vi "QueryFirst.vi"(6 "commandTimeout in":i32=-1, 7 "CommandType":i32(ring)=-1 items=["Text"=1, "StoredProcedure"=4, "TableDirect"=512], 8 "error in (no error)":errorcluster, 9 "DynamicParameters in":refnum<class "DynamicParameters.lvclass">, 10 "sql":string, 11 "SqlMapper in":refnum<class "DapperMapper.lvclass">) -> (0 "error out":errorcluster, 2 "Value":variant, 3 "SqlMapper out":refnum<class "DapperMapper.lvclass">)   [LabVIEW 2020, in "ORM_Dapper.lvlib" / "DapperMapper.lvclass"]
uses:
  DapperMapper.lvclass
  C:/Program Files/National Instruments/LabVIEW 2020/vi.lib/Viviota/shared/ORM.lvlibp/ORM/SqlMapper/SqlMapper.lvclass
  <vilib>/Viviota/shared/ORM.lvlibp/ORM/DynamicParameters/DynamicParameters.lvclass
  DapperParameters/DapperParameters.lvclass
  DapperRow/DapperRow.lvclass
  DapperParameters/DapperParameters.lvclass/DapperParameters.ctl
  C:/Viviota/Projects/R&D/LabVIEW_ORM/source/src/libraries/dapper/Dapper.dll
  libraries/dapper/Dapper.dll
  <vilib>/Viviota/shared/ORM.lvlibp/ORM/SqlMapper/Read DbConnection.vi
  <vilib>/Viviota/shared/ORM.lvlibp/ORM/DbConnection/Read connection.vi
  <vilib>/Viviota/shared/ORM.lvlibp/ORM/DbConnection/Read transaction.vi
  <vilib>/Viviota/shared/ORM.lvlibp/ORM/DbConnection/DbConnection.lvclass
  System.Data
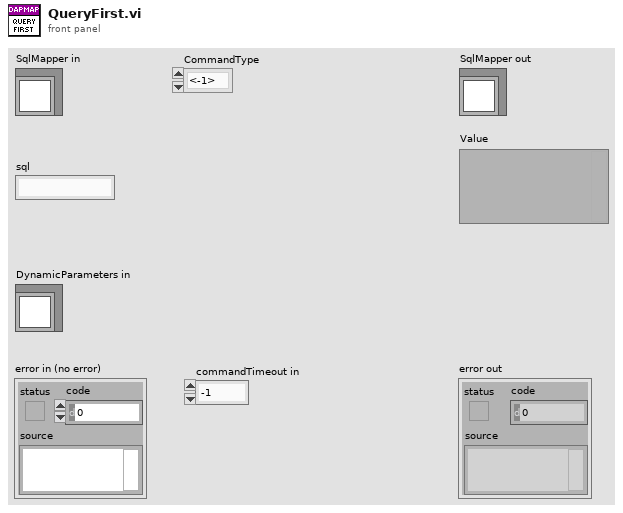
[diagram p1: front panel]
types:
  T1 = typedef "ORM_Dapper.lvlib/dapper_dynamicparameters_ref.ctl" = refnum<k24>
  T2 = typedef "ORM_Dapper.lvlib/dapper_sqlmapper_ref.ctl" = refnum<k24>
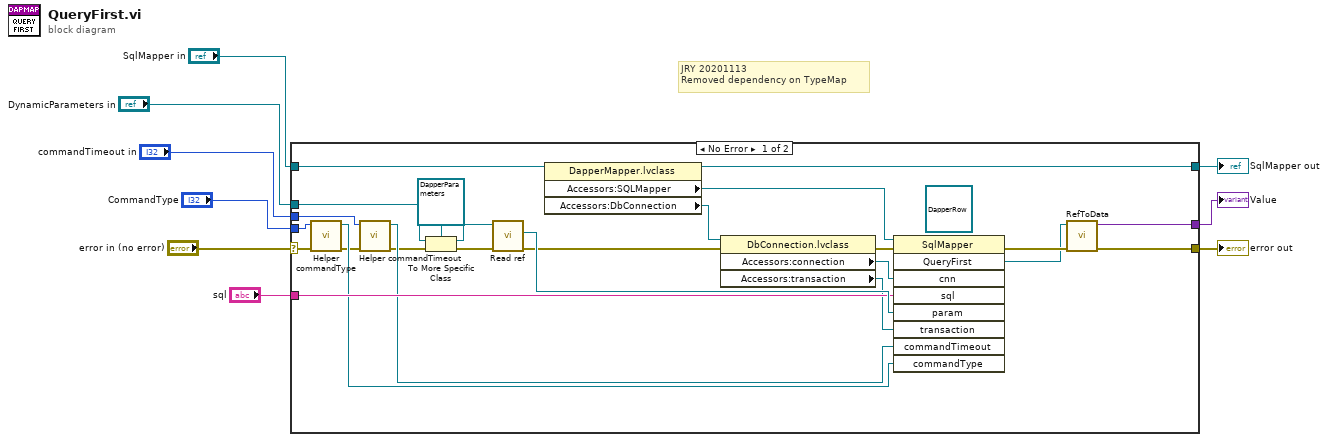
[diagram p0: block diagram]
diagram:
  # "JRY 20201113\nRemoved dependency on TypeMap"
  n1 = case shown="No Error" "error in (no error)" {
    selector: "error in (no error)" -> [w27 w36]
    tunnel: [w18 w36] -> w8
    tunnel: [w16 w35] -> w6
    tunnel: "SqlMapper in" -> [w30 w35]
    tunnel: "DynamicParameters in" -> [w12 _]
    tunnel: "sql" -> [w33 _]
    tunnel: "commandTimeout in" -> [w26 _]
    tunnel: "CommandType" -> [w25 _]
    tunnel: [w17 _] -> w1
    frame No Error {
      (unwired) refnum<class "DapperRow.lvclass"> refnum ("DapperRow in")
      n2 = call "Helper commandType.vi"("error in (no error)"=w27, "CommandType"=w25) -> ("error out"=w28:errorcluster, ".NET Refnum out"=w31:refnum<k24>)  [unwired: 8 in]
      n3 = call "Helper commandTimeout.vi"("error in (no error)"=w28, "commandTimeout in"=w26) -> ("error out"=w29:errorcluster, ".NET Refnum out"=w32:refnum<k24>)  [unwired: 8 in]
      n4 = To More Specific Class(target class=refnum<class "DapperParameters.lvclass"> refnum ("Dapper.lvlib:DynamicParameters"), reference=w12, error in=w29) -> (specific class reference=w11:refnum<class "DapperParameters.lvclass">, error out=w13:errorcluster)
      n5 = call "Read ref.vi"("error in (no error)"=w13, "DynamicParameters in"=w11) -> ("error out"=w22:errorcluster, "ref"=w34:T1)  [unwired: 7 in, 1 out]
      n6 = property class="DapperMapper.lvclass"(reference=w30) -> (reference out=w16:refnum<class "DapperMapper.lvclass">, "Accessors:SQLMapper"=w15:T2, "Accessors:DbConnection"=w14:refnum<class "DbConnection.lvclass">)  [unwired: 1 in, 1 out]
      n7 = property class="DbConnection.lvclass"(reference=w14, error in=w22) -> (error out=w21:errorcluster, "Accessors:connection"=w23:refnum<k24>, "Accessors:transaction"=w24:refnum<k24>)  [unwired: 1 out]
      n8 = invoke class="SqlMapper" method="QueryFirst"(reference=w15, error in=w21, "cnn"=w23, "sql"=w33, "param"=w34, "transaction"=w24, "commandTimeout"=w32, "commandType"=w31) -> (error out=w20:errorcluster, "QueryFirst"=w19:refnum<k24>)  [unwired: 1 in, 7 out]
      n9 = call "RefToData.vi"("error in (no error)"=w20, ".NET Refnum in"=w19) -> ("error out"=w18:errorcluster, "variant out"=w17:variant)  [unwired: 8 in]
    }
    frame Error {
    }
  }
  "error out" <- w8
  "SqlMapper out" <- w6
  "Value" <- w1
